vi "Select Random Value from Array.vi"(0 "Array":i32[](array[numeric])) -> (4 "Array Out":i32[](array[numeric]), 6 "Selected Value":i32, 8 "Selected Index":i32, 10 "Empty Array?":bool)   [LabVIEW 2014]
uses:
  Dragon Tamers.lvlib
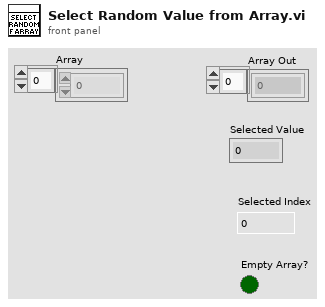
[diagram p1: front panel]
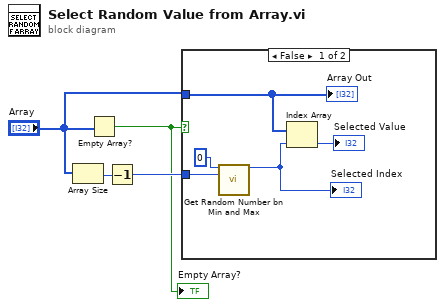
[diagram p0: block diagram]
diagram:
  n1 = Array Size(array="Array") -> (size(s)=w4:i32)
  n2 = Empty Array?(array="Array") -> (empty?=w1:bool)
  "Empty Array?" <- w1
  n3 = Decrement(x=w4) -> (x-1=w3:i32)
  n4 = case shown="False" w1 {
    tunnel: "Array" -> [w5 _]
    tunnel: w3 -> [w7 _]
    frame False {
      n5 = call "Get Random Number bn Min and Max.vi"("Min"=0, "Max"=w7) -> ("Random Value"=w8:i32)  [unwired: 13 in]
      "Selected Index" <- w8
      n6 = Index Array(array=w5, index=w8) -> (element=→"Selected Value":i32)
      "Array Out" <- w5
    }
    frame True {
    }
  }
